vi "PktToFrame.vi"(8 "FrameByte":u8, 9 "XORByte":u8, 10 "EscapeByte":u8, 11 "Packet":T1) -> (3 "Data":u8[](array[numeric]))   [LabVIEW 2009]
uses:
  Packet.ctl
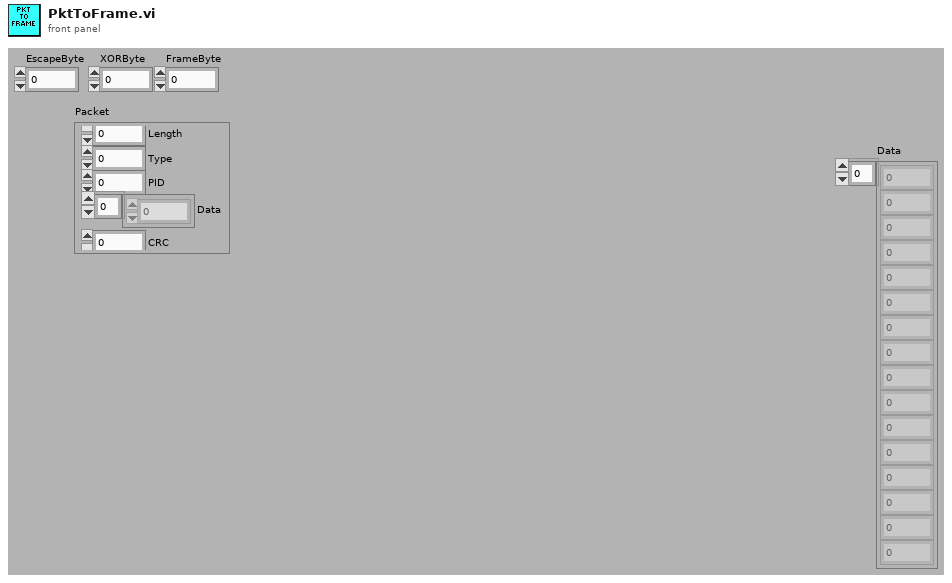
[diagram p1: front panel]
types:
  T1 = typedef "Packet.ctl" = cluster{"Length":u8, "Type":u8, "PID":u8, "Data":u8[], "CRC":u8}
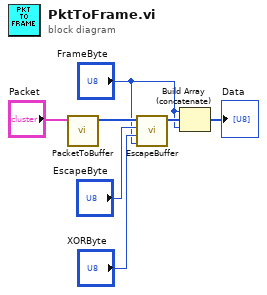
[diagram p0: block diagram]
diagram:
  n1 = call "PacketToBuffer.vi"("Packet"="Packet") -> ("Data"=w5:u8[])  [unwired: 10 in]
  n2 = call "EscapeBuffer.vi"("FrameByte"="FrameByte", "XORByte"="XORByte", "EscapeByte"="EscapeByte", "In"=w5) -> ("Out"=w2:u8[])  [unwired: 7 in]
  n3 = Build Array (concatenate)("FrameByte", w2, "FrameByte") -> (→"Data":u8[])
